vi "sequence util_findNreplace.vi"(8 "error in":errorcluster, 9 "Item Names IN":string[](array[string])=["----------    AH Bridge: Save GPIB address   ", "Write to VISA, GPIB::27::INSTR, FILE STORE GPIB USERPON", "----------    LakeShore 340 controller: change heater power (0-5, 0: off)  ", "Write to VISA, GPIB::12::INSTR, RANGE 0", "----------    Scheduled T-control for the He3 system   ", "Wait for 12 hour", "Set Temperature LS336 ( GPIB0::12::INSTR ) 45 K at 0 K/min, Output 1", "Wait for 60 s", "Wait for Temperature Less than 1.8 K Sensor C of LS336 ( GPIB0::14::INSTR ) Timeout 30 min", "Wait for 60 min", "Set Temperature LS336 ( GPIB0::12::INSTR ) 0.1 K at 0 K/min, Output 1", "----------    Motor control (use Instrumet:Set:MotorControl command structure)  ", "Set MotorControl ( BLM ) 12345 0.2", "Wait for VI value localhost, BLM_ManualControl.vi, BLM Position, Within, 12345, 10 min", "Wait for 10 s", "END SEQUENCE"], 11 "sequence in":string="----------    AH Bridge: Save GPIB address   \nWrite to VISA, GPIB::27::INSTR, FILE STORE GPIB USERPON\n----------    LakeShore 340 controller: change heater power (0-5, 0: off)  \nWrite to VISA, GPIB::12::INSTR, RANGE 0\n----------    Scheduled T-control for the He3 system   \nWait for 12 hour\nSet Temperature LS336 ( GPIB0::12::INSTR ) 45 K at 0 K/min, Output 1\nWait for 60 s\nWait for Temperature Less than 1.8 K Sensor C of LS336 ( GPIB0::14::INSTR ) Timeout 30 min\nWait for 60 min\nSet Temperature LS336 ( GPIB0::12::INSTR ) 0.1 K at 0 K/min, Output 1\n----------    Motor control (use Instrumet:Set:MotorControl command structure)  \nSet MotorControl ( BLM ) 12345 0.2\nWait for VI value localhost, BLM_ManualControl.vi, BLM Position, Within, 12345, 10 min\nWait for 10 s\nEND SEQUENCE") -> (0 "error out":errorcluster, 1 "Item Names out":string[](array[string])=["----------    AH Bridge: Save GPIB address   ", "Write to VISA, GPIB::27::INSTR, FILE STORE GPIB USERPON", "----------    LakeShore 340 controller: change heater power (0-5, 0: off)  ", "Write to VISA, GPIB::12::INSTR, RANGE 0", "----------    Scheduled T-control for the He3 system   ", "minsadfaf 12 hour", "Set Temperature LS336 ( GPIB0::12::INSTR ) 45 K at 0 K/min, Output 1", "minsadfaf 601 s", "minsadfaf Temperature Less than 1.8 K Sensor C of LS336 ( GPIB0::14::INSTR ) Timeout 30 min", "minsadfaf 601 min", "Set Temperature LS336 ( GPIB0::12::INSTR ) 0.1 K at 0 K/min, Output 1", "----------    Motor control (use Instrumet:Set:MotorControl command structure)  ", "Set MotorControl ( BLM ) 12345 0.2", "minsadfaf VI value localhost, BLM_ManualControl.vi, BLM Position, Within, 12345, 10 min", "minsadfaf 10 s", "END SEQUENCE"], 3 "sequence out":string="----------    AH Bridge: Save GPIB address   \nWrite to VISA, GPIB::27::INSTR, FILE STORE GPIB USERPON\n----------    LakeShore 340 controller: change heater power (0-5, 0: off)  \nWrite to VISA, GPIB::12::INSTR, RANGE 0\n----------    Scheduled T-control for the He3 system   \nminsadfaf 12 hour\nSet Temperature LS336 ( GPIB0::12::INSTR ) 45 K at 0 K/min, Output 1\nminsadfaf 601 s\nminsadfaf Temperature Less than 1.8 K Sensor C of LS336 ( GPIB0::14::INSTR ) Timeout 30 min\nminsadfaf 601 min\nSet Temperature LS336 ( GPIB0::12::INSTR ) 0.1 K at 0 K/min, Output 1\n----------    Motor control (use Instrumet:Set:MotorControl command structure)  \nSet MotorControl ( BLM ) 12345 0.2\nminsadfaf VI value localhost, BLM_ManualControl.vi, BLM Position, Within, 12345, 10 min\nminsadfaf 10 s\nEND SEQUENCE")   [LabVIEW 2025]
panel:
  in  "Cancel":bool
  in  "Execute?":bool
  in  "find and replace":T1(array[cluster])=[{"replace this"="Set Parameter", "with this"="Set Parameter localhost,"}, {"replace this"="Wait forTemperature", "with this"="Wait for VI value localhost,"}, {"replace this"="Wait for", "with this"="minsadfaf"}, {"replace this"="60", "with this"="601"}]
  # "1. Find and replace strings in the sequence.\n2. If executed, it will return the resulting sequence the host VI (sequence utility.vi)\n3. One can also accept or reject the change at the host VI (sequence utility.vi) level."
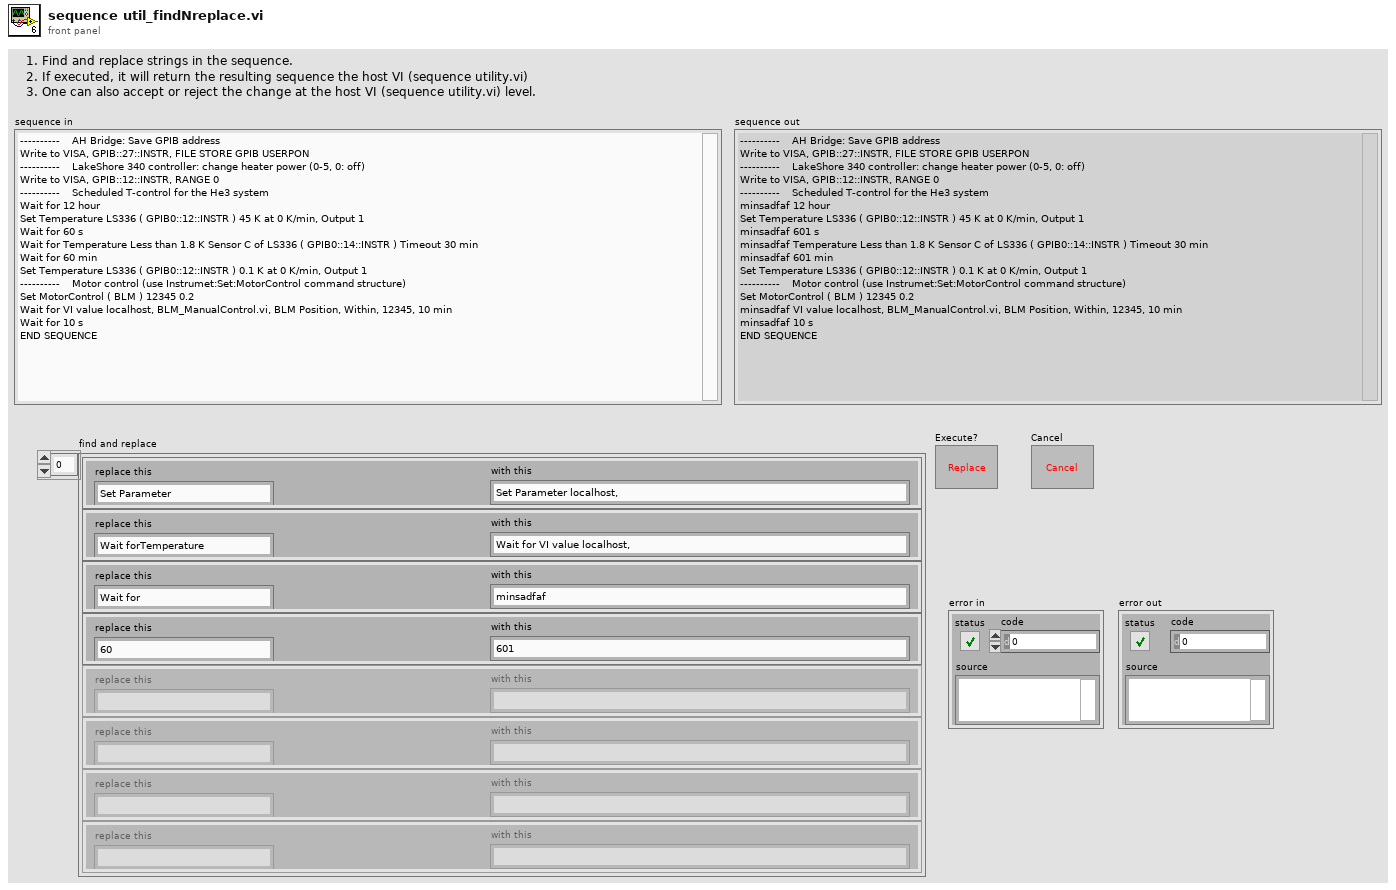
[diagram p1: front panel]
types:
  T1 = cluster{"replace this":string, "with this":string}[]
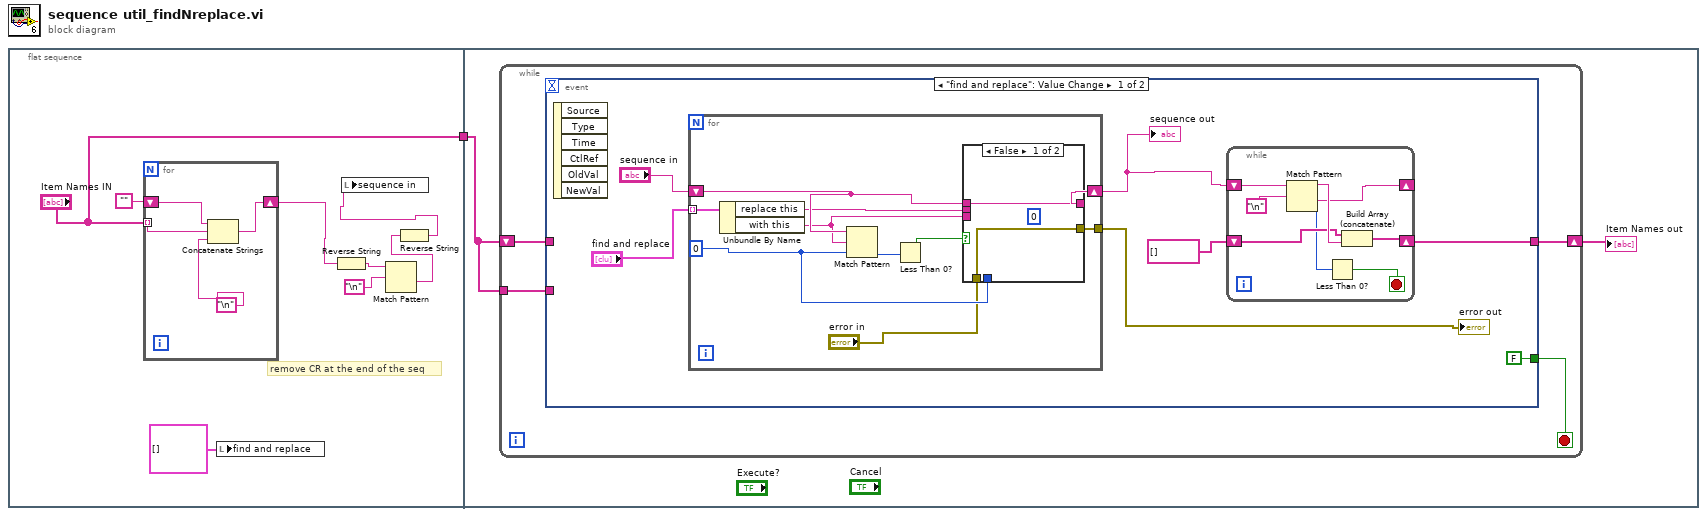
[diagram p0: block diagram]
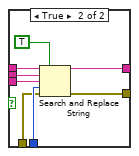
[diagram p2: hidden frame]
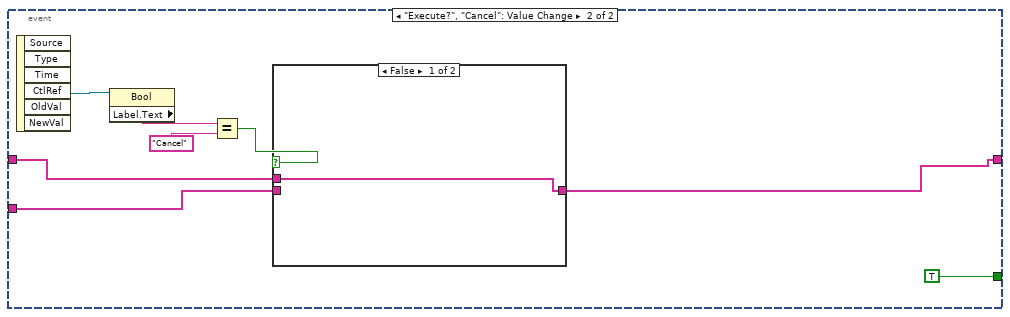
[diagram p3: hidden frame]
diagram:
  n1 = flat-sequence {
    tunnel: ["Item Names IN"] -> w1
    tunnel: w1 -> [w14]
    frame #0 {
      # "remove CR at the end of the seq"
      n2 = for {
        shift-right: [w12] -> w6
        shift-left: "" -> [w13]
        tunnel: "Item Names IN" -> [w11] mode=indexing
        n3 = Concatenate Strings(w13, w11, "\n") -> (w12:string)
      }
      n4 = local write "find and replace"(T1 [] ("find and replace")) -> ()
      n5 = Reverse String(1:w6) -> (0:w7:string)
      n6 = Match Pattern(string=w7, regular expression="\n") -> (after substring=w8:string)  [unwired: 1 in, 3 out]
      n7 = Reverse String(1:w8) -> (0:w9:string)
      n8 = local write "sequence in"(w9) -> ()
    }
    frame #1 {
      n9 = while {
        shift-right: [w18] -> w15
        shift-left: w14 -> [w17]
        tunnel: w14 -> [w16]
        stop <- w19 stop-if-true
        n10 = event shown="[0] \"find and replace\": Value Change" {
          selector: _ -> [_ _]
          dyn-events: _ -> [_ _]
          timeout: _ -> [_ _]
          tunnel: [FALSE TRUE] -> w19
          tunnel: [w20 w57] -> w18
          tunnel: w17 -> [_ w55]
          tunnel: w16 -> [_ w56]
          event "find and replace": Value Change {
            n11 = event-data() -> ()  [unwired: 1 in, 6 out]
            n12 = for {
              tunnel: "find and replace" -> [w44] mode=indexing
              shift-right: [w42] -> w23
              shift-left: "sequence in" -> [w43]
              tunnel: [w35] -> w22
              w40 = 0 ("offset past replacement")
              n13 = Unbundle By Name(w44) -> ("replace this"=w38:string, "with this"=w37:string)
              n14 = Match Pattern(string=w43, regular expression=w37, offset (0)=w40) -> (offset past match=w39:i32)  [unwired: 3 out]
              n15 = Less Than 0?(x=w39) -> (x < 0?=w41:bool)
              n16 = case shown="False" w41 {
                tunnel: w43 -> [w46 w54]
                tunnel: w38 -> [_ w53]
                tunnel: w37 -> [_ w52]
                tunnel: [w46 w51] -> w42
                tunnel: w40 -> [_ w50]
                tunnel: "error in" -> [w45 w48]
                tunnel: [w45 w47] -> w35
                frame False {
                  (unwired) 0 ("number of replacements")
                }
                frame True {
                  n17 = Search and Replace String(replace all?=TRUE ("replace all? (F)"), input string=w54, search string=w53, replace string=w52, offset=w50, error in=w48) -> (result string=w51:string, error out=w47:errorcluster)  [unwired: 2 in, 2 out]
                }
              }
            }
            "sequence out" <- w23
            "error out" <- w22
            n18 = while {
              shift-right: [w31] -> _
              shift-left: w23 -> [w34]
              shift-right: [w29] -> w20
              shift-left: string[] [] -> [w30]
              stop <- w27 stop-if-true
              n19 = Match Pattern(string=w34, regular expression="\n") -> (before substring=w32:string, after substring=w31:string, offset past match=w28:i32)  [unwired: 1 in, 1 out]
              n20 = Less Than 0?(x=w28) -> (x < 0?=w27:bool)
              n21 = Build Array (concatenate)(w30, w32) -> (w29:string[])
            }
          }
          event "Execute?", "Cancel": Value Change {
            n22 = event-data() -> ("CtlRef"=w61:refnum<vi>)  [unwired: 1 in, 5 out]
            n23 = property class="Bool"(reference=w61) -> ("Label.Text"=w60:string)  [unwired: 1 in, 2 out]
            n24 = Equal?(x=w60, y="Cancel" ("Label.Text")) -> (x = y?=w58:bool)
            n25 = case shown="False" w58 {
              tunnel: [w63 w64] -> w57
              tunnel: w56 -> [_ w64]
              tunnel: w55 -> [w63 _]
              frame False {
              }
              frame True {
              }
            }
          }
        }
      }
      "Item Names out" <- w15
    }
  }
